vi "Sort.vi"(8 "desend":bool, 10 "Array":string[](array[string])) -> (0 "sorted Index":i32[](array[numeric]), 2 "sorted":string[](array[string]))   [LabVIEW 2011]
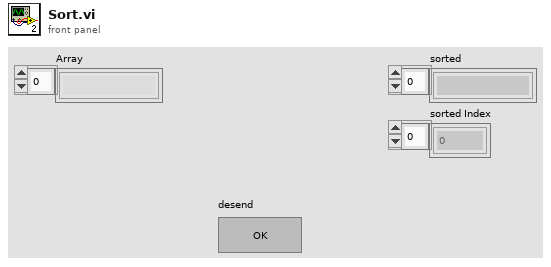
[diagram p1: front panel]
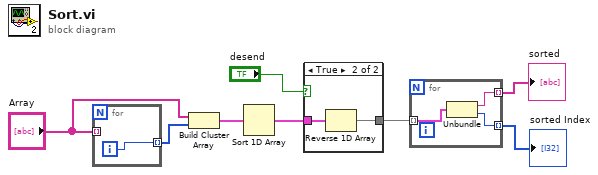
[diagram p0: block diagram]
diagram:
  n1 = for {
    tunnel: [w9] -> w8 mode=indexing
    tunnel: "Array" -> [_] mode=indexing
    i -> [w9]
  }
  n2 = Build Cluster Array("Array", w8) -> (w6:cluster{string, i32}[])
  n3 = Sort 1D Array(array=w6) -> (sorted array=w5:cluster{string, i32}[])
  n4 = case shown="True" "desend" {
    tunnel: w5 -> [w10 w12]
    tunnel: [w10 w11] -> w3
    frame False {
    }
    frame True {
      n5 = Reverse 1D Array(array=w12) -> (reversed array=w11:cluster{string, i32}[])
    }
  }
  n6 = for {
    tunnel: w3 -> [w15] mode=indexing
    tunnel: [w14] -> w2 mode=indexing
    tunnel: [w13] -> w1 mode=indexing
    n7 = Unbundle(w15) -> (w14:string, w13:i32)
  }
  "sorted" <- w2
  "sorted Index" <- w1
